vi "Try D-E Tovey Receive.vi"(8 "error in (no error)":errorcluster, 11 "Model in":refnum<class "Model.lvclass">) -> (0 "error out":errorcluster, 2 "Data Present":bool, 3 "Model out":refnum<class "Model.lvclass">)   [LabVIEW 2015, in "Model.lvclass"]
uses:
  Model.lvclass
  Model.lvclass/Model.ctl
  TEI-9150/Tovey 9150.lvclass
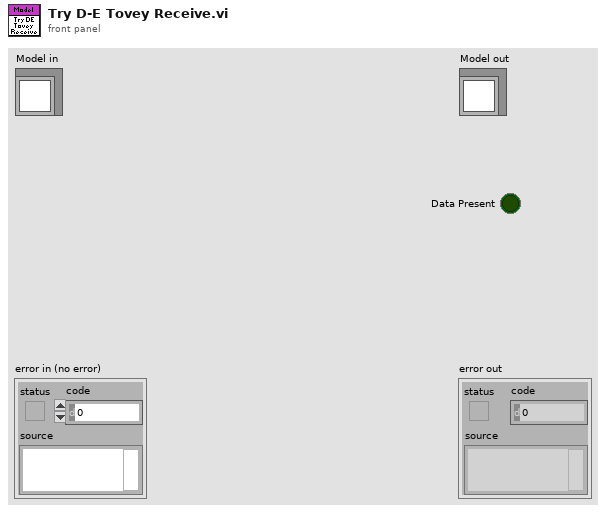
[diagram p1: front panel]
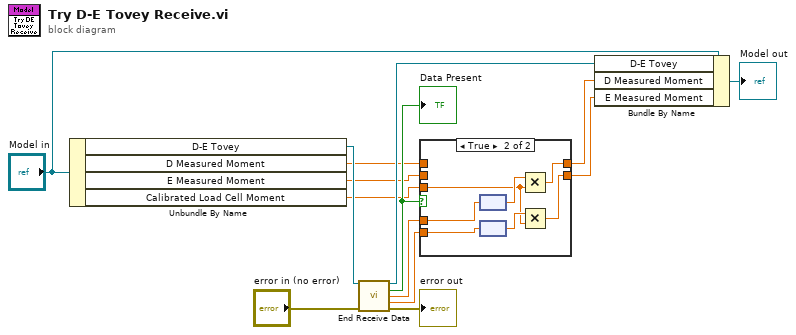
[diagram p0: block diagram]
diagram:
  n1 = Unbundle By Name("Model in") -> ("D-E Tovey"=w12:refnum<class "Tovey 9150.lvclass">, "D Measured Moment"=w9:dbl[unit], "E Measured Moment"=w7:dbl[unit], "Calibrated Load Cell Moment"=w1:dbl[unit])
  n2 = call "End Receive Data.vi"("Tovey9150 in"=w12, "error in (no error)"="error in (no error)") -> ("Tovey9150 out"=w11:refnum<class "Tovey 9150.lvclass">, "Data Present"=w10:bool, "A"=w5:dbl, "B"=w4:dbl, "error out"=→"error out":errorcluster)  [unwired: 9 in]
  "Data Present" <- w10
  n3 = case shown="True" w10 {
    tunnel: w9 -> [w16 _]
    tunnel: [w16 w19] -> w8
    tunnel: w7 -> [w15 _]
    tunnel: [w15 w18] -> w6
    tunnel: w5 -> [_ w23]
    tunnel: w4 -> [_ w22]
    tunnel: w1 -> [_ w17]
    frame False {
    }
    frame True {
      n4 = node(w23) -> (w20:dbl[unit])
      n5 = node(w22) -> (w21:dbl[unit])
      n6 = Multiply(x=w20, y=w17) -> (x*y=w19:dbl[unit])
      n7 = Multiply(x=w21, y=w17) -> (x*y=w18:dbl[unit])
    }
  }
  n8 = Bundle By Name(cluster="Model in", "D-E Tovey"=w11, "D Measured Moment"=w8, "E Measured Moment"=w6) -> (→"Model out":refnum<class "Model.lvclass">)
